vi "Process.vi"(0 "reference in":refnum<class "active object queue.lvclass">, 5 "error in (no error)":errorcluster) -> (14 "reference out":refnum<class "active object queue.lvclass">, 19 "error out":errorcluster)   [LabVIEW 2019, in "active object queue.lvclass"]
uses:
  active object queue.lvclass
  <vilib>/Platform/TimedLoop/XDataNode/timing_clust.ctl
  <vilib>/Platform/TimedLoop/XDataNode/nitl_modes.ctl
  <vilib>/Platform/TimedLoop/XDataNode/wakeup.ctl
  <vilib>/platform/TimedLoop/XDataNode/XDataNode.xnode
  <vilib>/Platform/TimedLoop/XDataNode/XDNodeRunTimeDep.lvlib
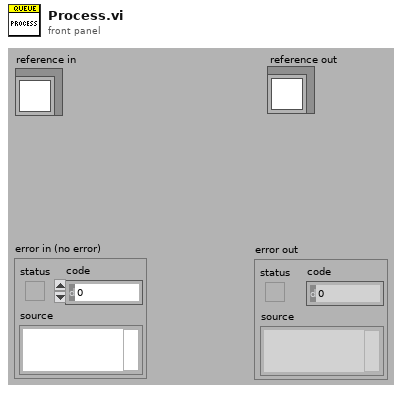
[diagram p1: front panel]
types:
  T1 = typedef "XDNodeRunTimeDep.lvlib/timing_clust.ctl" = cluster{"Expected End [f-1]":u64, "Actual End [f-1]":u64, "Finished Late? [f-1]":bool, "Expected End [i-1]":u64, "Actual End [i-1]":u64, "Finished Late? [i-1]":bool, "Expected Start [i]":u64, "Actual Start [i]":u64, "Expected Start [f]":u64, "Actual Start [f]":u64, "Source Name":string, "Structure Name":string, "Period":i64, "Deadline":i64, "Offset":i64, "Start":i64, "Priority":i32, "Timeout":i32, "Mode":T2, "Wakeup Reason":T3, "Error":errorcluster, "Source Type":string, "Secondary Source Type":string, "Global End Time":u64, "Global Start Time":u64, "Frame Duration":u64, "Iteration Duration":u64, "Assigned CPU":i32, "I/O Scan Engine Mode":u32}
  T2 = typedef "XDNodeRunTimeDep.lvlib/nitl_modes.ctl" = enum32{"No Change", "Process missed periods, maintain original phase", "Discard missed periods, maintain original phase", "Process missed periods, ignore original phase", "Discard missed periods, ignore original phase"}
  T3 = typedef "XDNodeRunTimeDep.lvlib/wakeup.ctl" = enum32{"Normal", "Aborted", "Asynchronous wakeup", "Timing source error", "Timed loop error", "Timeout"}
  T4 = typedef "active object queue.lvclass/ObjectAttributes.ctl" = cluster{"Attribute1":dbl, "Status":bool}
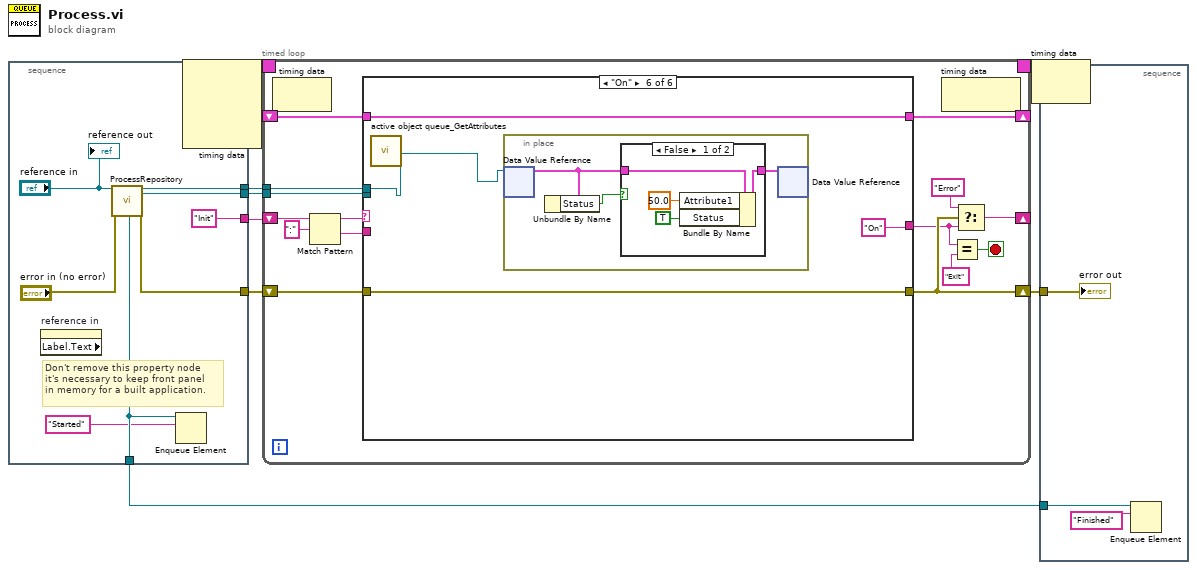
[diagram p0: block diagram]
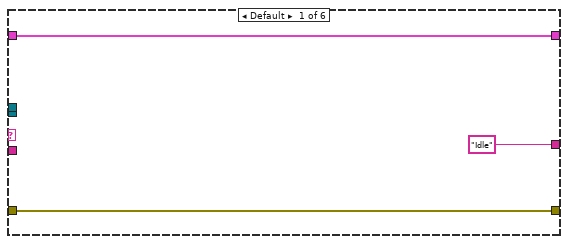
[diagram p2: hidden frame]
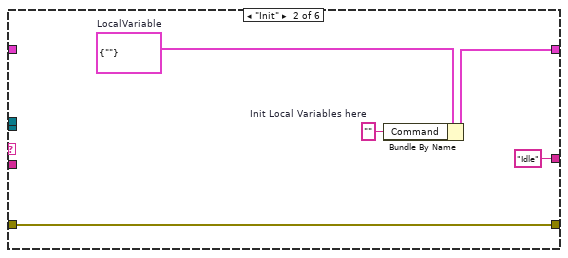
[diagram p3: hidden frame]
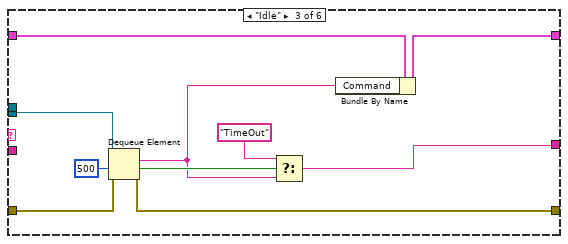
[diagram p4: hidden frame]
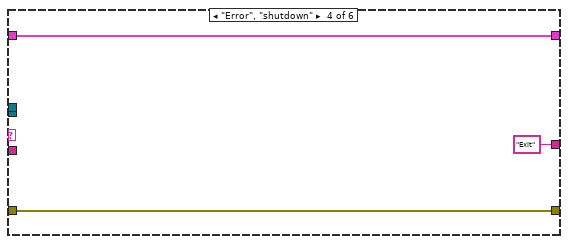
[diagram p5: hidden frame]
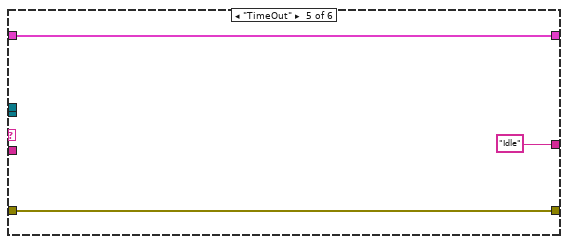
[diagram p6: hidden frame]
diagram:
  n1 = stacked-sequence {
    tunnel: [w13] -> w8
    tunnel: [w16] -> w6
    tunnel: [w12] -> w5
    tunnel: [w10] -> w4
    tunnel: ["Init"] -> w3
    frame #0 {
      # "Don't remove this property node\nit's necessary to keep front panel\nin memory for a built application."
      n2 = property on="reference in" class="LVClassControl (strict)" props=["Label", "Text"]() -> ()  [unwired: 2 in, 3 out]
      n3 = call "ProcessRepository.vi"("reference in"="reference in", "error in (no error)"="error in (no error)") -> ("ProcessSyncQueue"=w10:refnum<queue>, "reference out"=w16:refnum<class "active object queue.lvclass">, "ToProcessQueue"=w12:refnum<queue>, "error out"=w13:errorcluster)  [unwired: 11 in, 3 out]
      n4 = Enqueue Element(queue=w10, element="Started") -> ()  [unwired: 2 in, 3 out]
      "reference out" <- "reference in"
    }
  }
  n5 = node-c288() -> (w2:T1)  [unwired: 4 in]
  n6 = timed-loop {
    shift-right: [w24] -> w7
    shift-left: w8 -> [w29]
    tunnel: w6 -> [w30]
    tunnel: w5 -> [w31]
    shift-right: [w22] -> _
    shift-left: w3 -> [w27]
    shift-right: [w18] -> _
    shift-left: _ -> [w17]
    timing: w2 -> [_]
    timing-out: [_] -> w1
    stop <- w19 stop-if-true
    n7 = node-c288() -> ()  [unwired: 1 in, 1 out]
    n8 = Match Pattern(string=w27, regular expression=":") -> (before substring=w26:string, after substring=w25:string)  [unwired: 1 in, 2 out]
    n9 = case shown="\"On\"" w26 {
      tunnel: w29 -> [w36 w38 w49 w54 w57 w60]
      tunnel: [w36 w38 w48 w54 w57 w60] -> w24
      tunnel: w31 -> [_ _ w50 _ _ _]
      tunnel: w30 -> [_ _ _ _ _ w62]
      tunnel: w25 -> [_ _ _ _ _ _]
      tunnel: ["Idle" ("t") "Idle" ("t") w45 "Exit" ("y") "Idle" ("t") "On" ("t")] -> w21
      tunnel: [w34 w40 w42 w52 w55 w61] -> w18
      tunnel: w17 -> [w34 _ w43 w52 w55 w61]
      frame Default {
      }
      frame "Init" {
        w39 = ""  # Init Local Variables here
        w41 = cluster{"Command":string} {"Command"=""}  # LocalVariable
        n10 = Bundle By Name(cluster=w41, "Command"=w39) -> (w40:cluster{"Command":string})
      }
      frame "Idle" {
        n11 = Dequeue Element(queue=w50, timeout in ms (-1)=500, error in (no error)=w49) -> (element=w44:string, timed out?=w47:bool, error out=w48:errorcluster)  [unwired: 1 out]
        n12 = Select(t="TimeOut", s=w47, f=w44) -> (s? t:f=w45:string)
        n13 = Bundle By Name(cluster=w43, "Command"=w44) -> (w42:cluster{"Command":string})
      }
      frame "Error", "shutdown" {
      }
      frame "TimeOut" {
      }
      frame "On" {
        n14 = call "active object queue_GetAttributes.vi"("reference in"=w62) -> ("DataRef"=w58:refnum<data-value>)  [unwired: 15 in, 3 out]
        n15 = in-place {
          n16 = in-place-dvr #1(w58) -> (w63:T4)  [unwired: 1 out]
          n17 = Unbundle By Name(w63) -> ("Status"=w64:bool)
          n18 = case shown="False" w64 {
            tunnel: [w69 w70] -> w65
            tunnel: w63 -> [w68 w70]
            frame False {
              n19 = Bundle By Name(cluster=w68, "Attribute1"=50.0, "Status"=TRUE) -> (w69:T4)
            }
            frame True {
            }
          }
          n20 = in-place-dvr #1(w65) -> ()  [unwired: 2 out]
        }
      }
    }
    n21 = node-c288() -> ()  [unwired: 1 in, 1 out]
    n22 = Equal?(x=w21, y="Exit") -> (x = y?=w19:bool)
    n23 = Select(t="Error", s=w24, f=w21) -> (s? t:f=w22:string)
  }
  n24 = node-c288(w1) -> ()  [unwired: 1 out]
  n25 = stacked-sequence {
    tunnel: w7 -> [w73]
    tunnel: w4 -> [w72]
    frame #0 {
      n26 = Enqueue Element(queue=w72, element="Finished") -> ()  [unwired: 2 in, 3 out]
      "error out" <- w73
    }
  }
